vi "Player Info.vi"(11 "Net in":refnum<class "Net.lvclass">) -> (1 "Victory Speech":string, 2 "Name":string, 3 "Net out":refnum<class "Net.lvclass">)   [LabVIEW 2015, in "Net.lvclass"]
uses:
  Net.lvclass
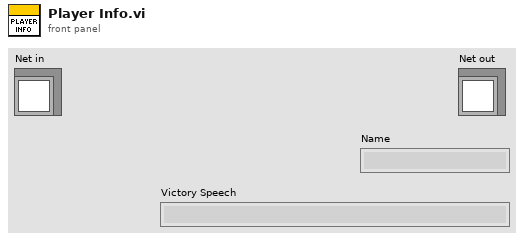
[diagram p1: front panel]
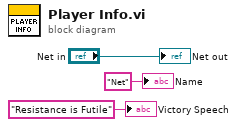
[diagram p0: block diagram]
diagram:
  "Net out" <- "Net in"
  "Name" <- "Net" ("Name")
  "Victory Speech" <- "Resistance is Futile" ("Victory Speech")
